vi "test图层.vi"() -> ()   [LabVIEW 2018]
doc: "This example demonstrates the use of binary morphological reconstruction in the particle analysis. The example allows you to keep the particles completely inside the ROI, completely outside the ROI or on the ROI."
uses:
  <vilib>/vision/NI_Vision_Development_Module.lvlib
panel:
  out "框组":T1(array[cluster])
  in  "单次删除":bool
  in  "Operation":T2(ring)
  out "重组图":T3(plugin-control)
  out "Image":T3(plugin-control)
  in  "Stop":bool
  # "Overview: Demonstrate the use of the Binary Morphology Reconstruction feature of Vision Development Module.\nRequirements: Vision Development Module.\nInstructions:\n1. Run the VI.\n2. Select the ROI in which you want to filter the objects. Press the <Ctrl> key to select multiple ROIs. \n3. Choose the required \"Operation\".\n  - Inner particles: Keeps all the particles completely inside the ROI.\n  - Outer particles: Keeps the particles completely outside the ROI.\n  - Boundary particles: Keeps the particles which are touching the boundary."
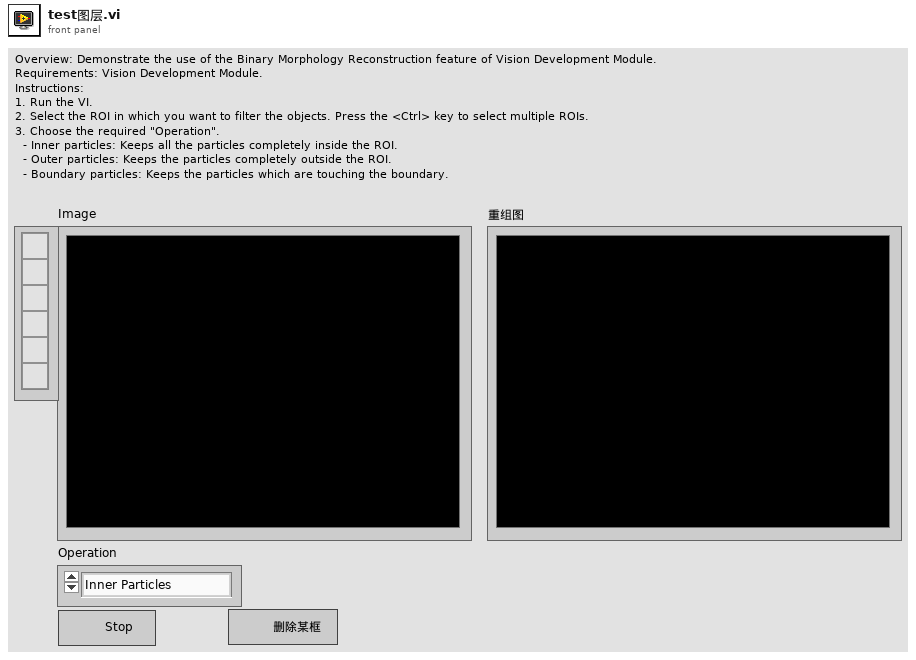
[diagram p1: front panel]
types:
  T1 = cluster{"Global Rectangle":i32[], "Contours":cluster{"Contour Type":u32, "ROI Type":u32, "Points":i32[]}[]}[]
  T2 = enum16{"Inner Particles", "Outer Particles", "Boundary Particles", "overlay rectangle"}
  T3 = typedef "IMAQ Image.ctl" = refnum<image>
  T4 = typedef "Image Type" = u32
  T5 = cluster{"Global Rectangle":i32[], "Contours":cluster{"Contour Type":u32, "ROI Type":u32, "Points":i32[]}[]}
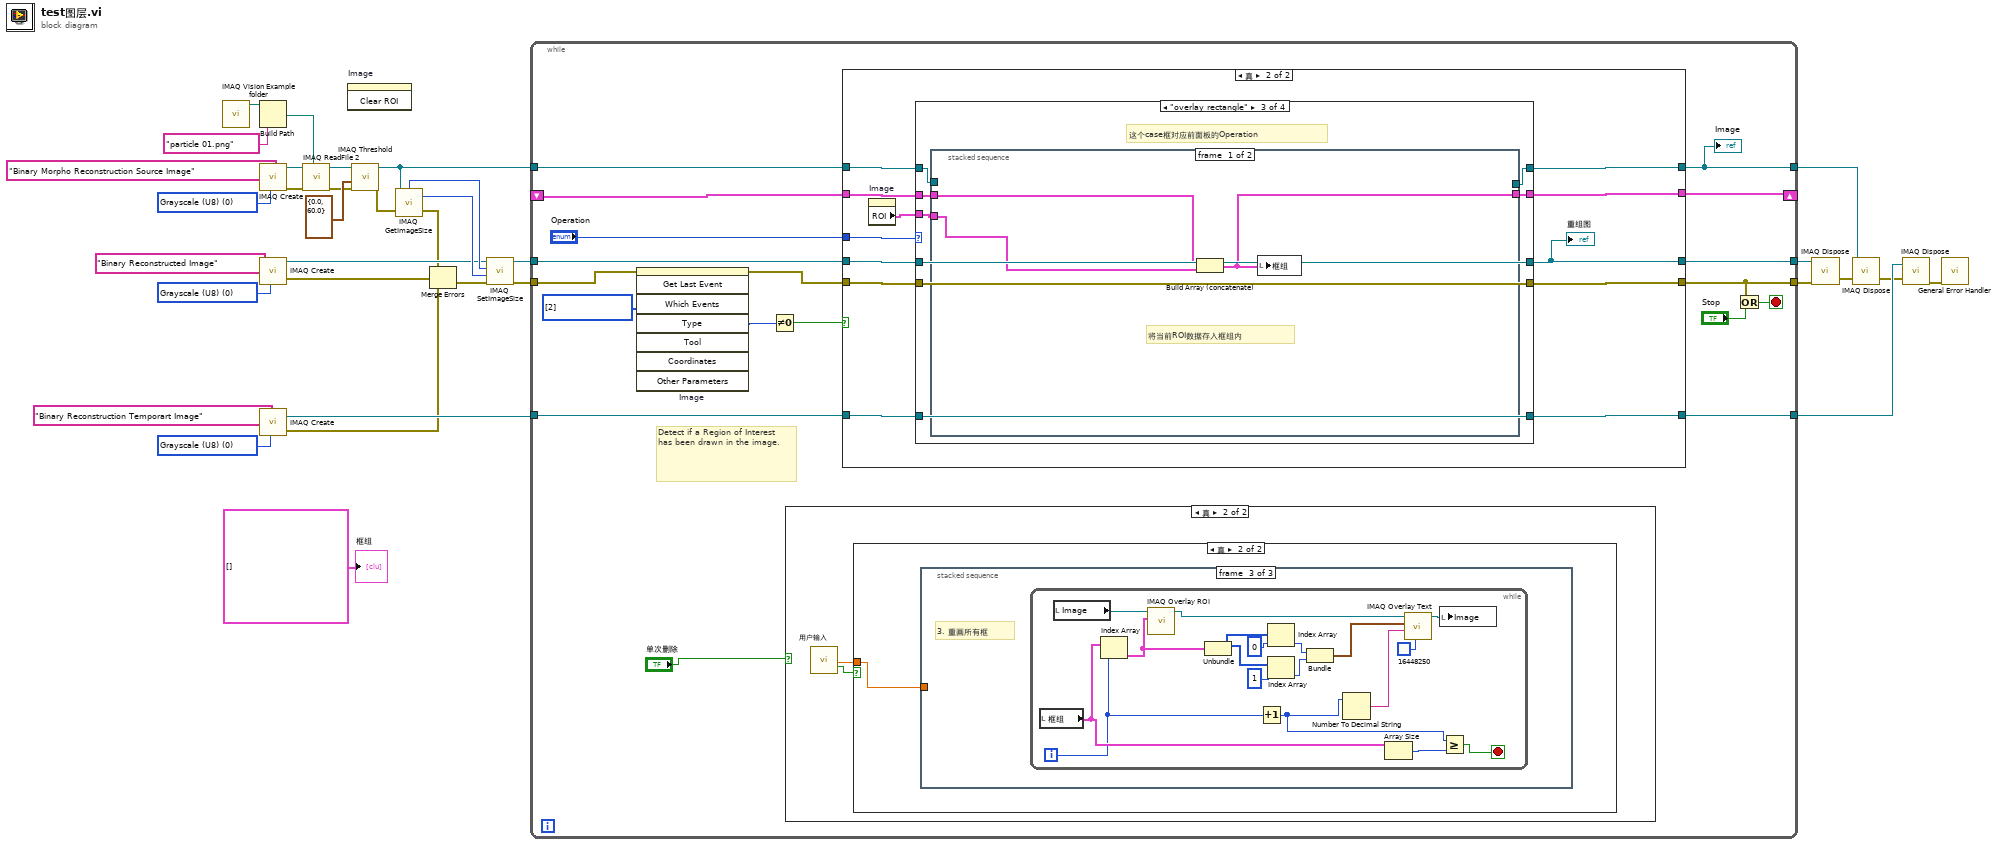
[diagram p0: block diagram]
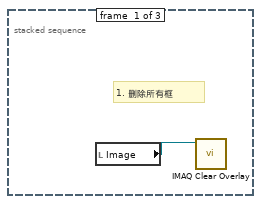
[diagram p4: hidden frame]
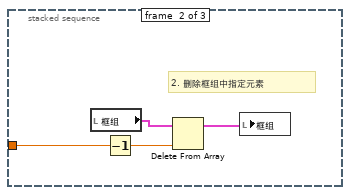
[diagram p5: hidden frame]
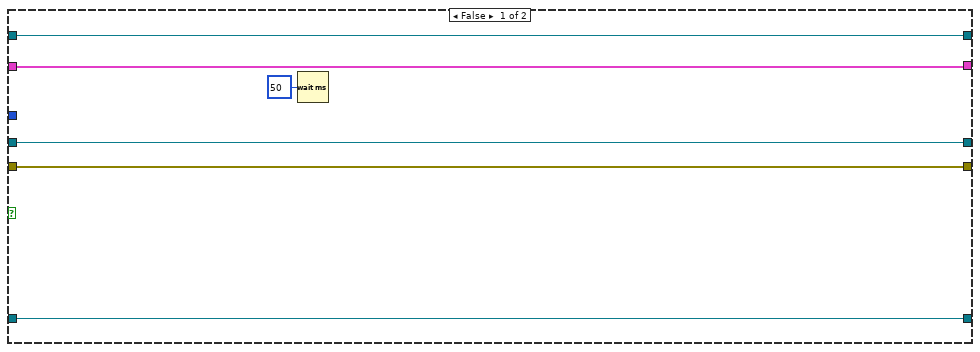
[diagram p6: hidden frame]
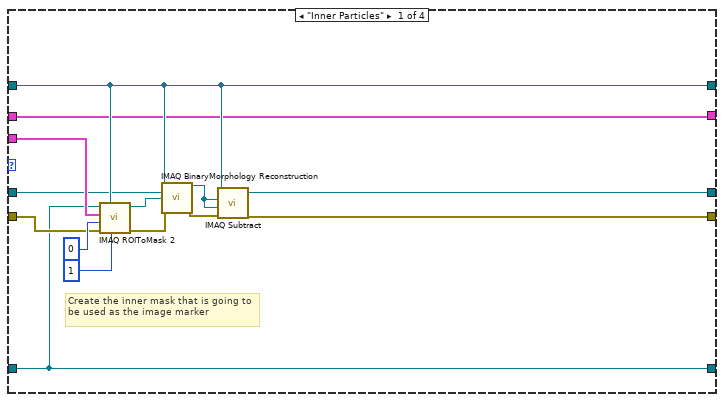
[diagram p7: hidden frame]
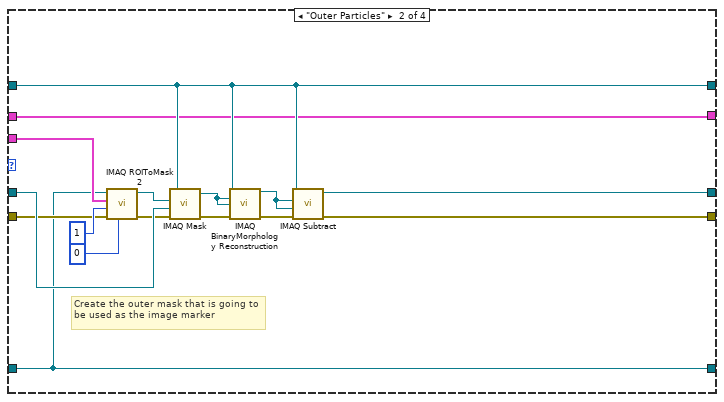
[diagram p8: hidden frame]
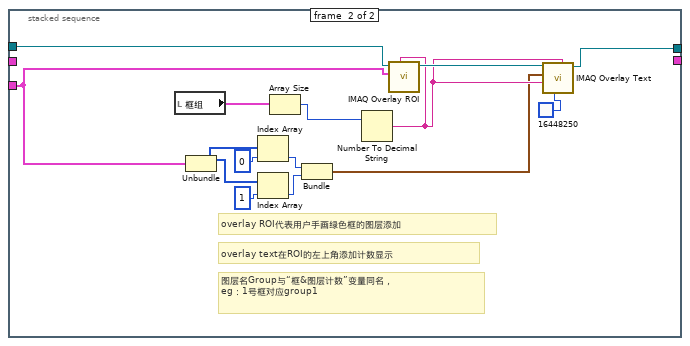
[diagram p9: hidden frame]
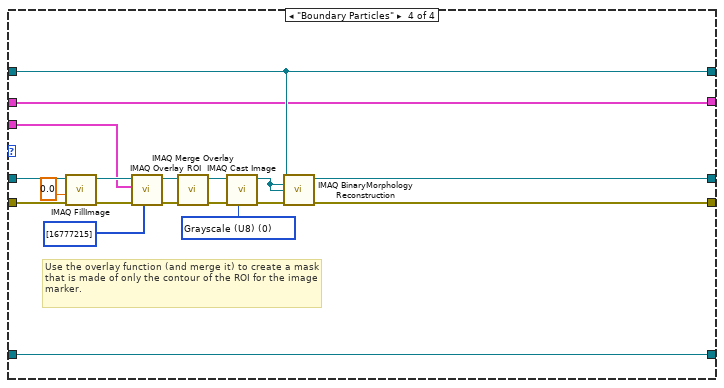
[diagram p10: hidden frame]
diagram:
  w24 = T4 0 items=["Grayscale (U8)", "Grayscale (I16)", "Grayscale (SGL)", "Complex (CSG)", "RGB (U32)", "HSL (U32)", "RGB (U64)", "Grayscale (U16)"] ("Image Type")
  w26 = T4 0 items=["Grayscale (U8)", "Grayscale (I16)", "Grayscale (SGL)", "Complex (CSG)", "RGB (U32)", "HSL (U32)", "RGB (U64)", "Grayscale (U16)"] ("Image Type")
  w27 = T4 0 items=["Grayscale (U8)", "Grayscale (I16)", "Grayscale (SGL)", "Complex (CSG)", "RGB (U32)", "HSL (U32)", "RGB (U64)", "Grayscale (U16)"] ("Image Type")
  n1 = call "IMAQ Vision Example folder.vi"() -> ("Example Image Path"=w33:path)  [unwired: 11 in]
  n2 = Build Path(base path=w33, name or relative path="particle 01.png") -> (appended path=w3:path)
  n3 = call "IMAQ Create"("Image Name"="Binary Morpho Reconstruction Source Image", "Image Type"=w26) -> ("New Image"=w30:T3, "error out"=w16:errorcluster)  [unwired: 2 in, 1 out]
  n4 = call "IMAQ Create"("Image Name"="Binary Reconstructed Image", "Image Type"=w27) -> ("New Image"=w20:T3, "error out"=w13:errorcluster)  [unwired: 2 in, 1 out]
  n5 = call "IMAQ Create"("Image Name"="Binary Reconstruction Temporart Image", "Image Type"=w24) -> ("New Image"=w21:T3, "error out"=w12:errorcluster)  [unwired: 2 in, 1 out]
  n6 = call "IMAQ ReadFile 2"("File Path"=w3, "error in (no error)"=w16, "Image"=w30) -> ("error out"=w15:errorcluster, "Image Out"=w18:T3)  [unwired: 4 in, 3 out]
  n7 = invoke on="Image" class="ImageControl" method="Clear ROI"() -> ()  [unwired: 3 in, 3 out]
  n8 = call "IMAQ Threshold"("error in (no error)"=w15, "Range"=cluster{"Lower value":sgl, "Upper value":sgl} {"Lower value"=0.0, "Upper value"=60.0}, "Image Src"=w18) -> ("error out"=w14:errorcluster, "Image Dst Out"=w2:T3)  [unwired: 3 in, 4 out]
  n9 = call "IMAQ GetImageSize"("Image"=w2, "error in (no error)"=w14) -> ("Y Resolution"=w22:i32, "X Resolution"=w23:i32, "error out"=w9:errorcluster)  [unwired: 2 out]
  n10 = Merge Errors(w9, w13, w12) -> (w11:errorcluster)
  n11 = call "IMAQ SetImageSize"("error in (no error)"=w11, "Y Resolution"=w22, "X Resolution"=w23, "Image"=w20) -> ("error out"=w10:errorcluster, "Image Out"=w19:T3)  [unwired: 1 out]
  n12 = while {
    tunnel: w2 -> [w52]
    tunnel: w19 -> [w51]
    tunnel: [w50] -> w29
    tunnel: [w39] -> w28
    tunnel: w21 -> [w49]
    tunnel: w10 -> [w45]
    tunnel: [w42] -> w7
    tunnel: [w43] -> w8
    shift-right: [w36] -> _
    shift-left: _ -> [w35]
    stop <- w40 stop-if-true
    w46 = i32[] [2] items=["No Event"=0, "Click Event"=1, "Draw Event"=2, "Size Event"=4, "Scroll Event"=5, "Double Click Event"=8] ("Which Events")
    # "Detect if a Region of Interest has been drawn in the image."
    n13 = invoke on="Image" class="ImageControl" method="Get Last Event"(error in=w45, "Which Events"=w46) -> (error out=w44:errorcluster, "Type"=w47:i32)  [unwired: 6 in, 6 out]
    n14 = Not Equal To 0?(x=w47) -> (x != 0?=w37:bool)
    n15 = case shown="真" "单次删除" {
      frame False {
      }
      frame True {
        n16 = call "用户输入"() -> ("框号"=w53:dbl, "确定"=w54:bool)  [unwired: 17 in, 1 out]
        n17 = case shown="真" w54 {
          tunnel: w53 -> [_ w55]
          frame False {
            # "用户取消操作"
          }
          frame True {
            n18 = stacked-sequence {
              tunnel: w55 -> [_ w59 _]
              frame #0 {
                # "1. 删除所有框"
                n19 = local read "Image"() -> (w56:T3)
                n20 = call "IMAQ Clear Overlay"("Image"=w56) -> ()  [unwired: 9 in, 2 out]
              }
              frame #1 {
                # "2. 删除框组中指定元素"
                n21 = local read "框组"() -> (w60:T1)
                n22 = Decrement(x=w59) -> (x-1=w58:dbl)
                n23 = Delete From Array(array=w60, index=w58) -> (array with subset deleted=w57:T1)  [unwired: 1 in, 1 out]
                n24 = local write "框组"(w57) -> ()
              }
              frame #2 {
                # "3. 重画所有框"
                n25 = while {
                  i -> [w68]
                  stop <- w77 stop-if-true
                  n26 = local read "框组"() -> (w69:T1)
                  n27 = local read "Image"() -> (w75:T3)
                  n28 = Index Array(array=w69, index=w68) -> (element=w63:T5)
                  n29 = call "IMAQ Overlay ROI"("ROI Descriptor"=w63, "Image"=w75) -> ("Image Out"=w71:T3)  [unwired: 8 in, 1 out]
                  n30 = Unbundle(w63) -> ("Global Rectangle"=w64:i32[])  [unwired: 1 out]
                  n31 = Increment(x=w68) -> (x+1=w74:i32)
                  n32 = Index Array(array=w64, index=0 ("索引")) -> (element=w65:i32)
                  n33 = Index Array(array=w64, index=1 ("索引")) -> (element=w66:i32)
                  n34 = Bundle(w65, w66) -> (w62:cluster{i32, i32})  [unwired: 1 in]
                  n35 = Number To Decimal String(number=w74) -> (decimal integer string=w72:string)  [unwired: 1 in]
                  n36 = Array Size(array=w69) -> (size(s)=w76:i32)
                  n37 = call "IMAQ Overlay Text"("Text Color (black)"=u32 16448250, "String"=w72, "Origin"=w62, "Image"=w71) -> ("Image Out"=w70:T3)  [unwired: 6 in, 1 out]
                  n38 = local write "Image"(w70) -> ()
                  n39 = Greater Or Equal?(x=w74, y=w76) -> (x >= y?=w77:bool)
                }
              }
            }
          }
        }
      }
    }
    n40 = case shown="真" w37 {
      tunnel: w52 -> [w83 w95]
      tunnel: w51 -> [w82 w94]
      tunnel: [w82 w93] -> w50
      tunnel: [w83 w92] -> w39
      tunnel: w49 -> [w80 w87]
      tunnel: "Operation" -> [_ w90]
      tunnel: w44 -> [w81 w89]
      tunnel: [w81 w88] -> w42
      tunnel: [w80 w86] -> w43
      tunnel: [w78 w85] -> w36
      tunnel: w35 -> [w78 w84]
      frame False {
        n41 = Wait (ms)(milliseconds to wait=u32 50) -> ()  [unwired: 1 out]
      }
      frame True {
        n42 = property on="Image" class="ImageControl"() -> ("ROI"=w91:T5)  [unwired: 2 in, 2 out]
        n43 = case shown="\"overlay rectangle\"" w90 {
          tunnel: w95 -> [w104 w117 w130 w166]
          tunnel: w94 -> [w102 w118 w133 w158]
          tunnel: w87 -> [w97 w111 w131 w167]
          tunnel: [w106 w120 w133 w169] -> w93
          tunnel: w91 -> [w105 w119 w128 w159]
          tunnel: [w104 w117 w129 w166] -> w92
          tunnel: w89 -> [w101 w116 w132 w157]
          tunnel: [w98 w112 w132 w168] -> w88
          tunnel: [w97 w111 w131 w167] -> w86
          tunnel: [w96 w110 w127 w151] -> w85
          tunnel: w84 -> [w96 w110 w126 w151]
          frame "Inner Particles" {
            # "Create the inner mask that is going to be used as the image marker"
            n44 = call "IMAQ ROIToMask 2"("Background Value (0)"=1, "Image Model"=w104, "error in (no error)"=w101, "Filling Value (255)"=0, "ROI Descriptor"=w105, "Image"=w97) -> ("error out"=w100:errorcluster, "Image Out"=w103:T3)  [unwired: 4 out]
            n45 = call "IMAQ BinaryMorphology Reconstruction"("Image Src"=w104, "Image Dst"=w102, "Image Marker"=w103, "error in (no error)"=w100) -> ("Image Dst Out"=w107:T3, "error out"=w99:errorcluster)  [unwired: 4 in, 6 out]
            n46 = call "IMAQ Subtract"("Image Src A"=w104, "Image Dst"=w107, "Image Src B"=w107, "error in (no error)"=w99) -> ("Image Dst Out"=w106:T3, "error out"=w98:errorcluster)  [unwired: 1 in, 2 out]
          }
          frame "Outer Particles" {
            # "Create the outer mask that is going to be used as the image marker"
            n47 = call "IMAQ ROIToMask 2"("Background Value (0)"=0, "error in (no error)"=w116, "Filling Value (255)"=1, "ROI Descriptor"=w119, "Image"=w111) -> ("error out"=w115:errorcluster, "Image Out"=w123:T3)  [unwired: 1 in, 4 out]
            n48 = call "IMAQ Mask"("error in (no error)"=w115, "Image Dst"=w118, "Image Mask"=w123, "Image Src"=w117) -> ("error out"=w114:errorcluster, "Image Dst Out"=w122:T3)  [unwired: 1 out]
            n49 = call "IMAQ BinaryMorphology Reconstruction"("Image Src"=w117, "Image Dst"=w122, "Image Marker"=w122, "error in (no error)"=w114) -> ("Image Dst Out"=w121:T3, "error out"=w113:errorcluster)  [unwired: 4 in, 6 out]
            n50 = call "IMAQ Subtract"("Image Src A"=w117, "Image Dst"=w121, "Image Src B"=w121, "error in (no error)"=w113) -> ("Image Dst Out"=w120:T3, "error out"=w112:errorcluster)  [unwired: 1 in, 2 out]
          }
          frame "overlay rectangle" {
            # "这个case框对应前面板的Operation"
            n51 = stacked-sequence {
              tunnel: w130 -> [_ w140]
              tunnel: [_ w139] -> w129
              tunnel: w128 -> [w136 w141]
              tunnel: [w134 _] -> w127
              tunnel: w126 -> [w135 _]
              frame #0 {
                # "将当前ROI数据存入框组内"
                n52 = Build Array (concatenate)(w135, w136) -> (w134:T1)
                n53 = local write "框组"(w134) -> ()
              }
              frame #1 {
                # "图层名Group与“框&图层计数”变量同名，\neg：1号框对应group1"
                # "overlay text在ROI的左上角添加计数显示"
                # "overlay ROI代表用户手画绿色框的图层添加"
                n54 = local read "框组"() -> (w146:T1)
                n55 = Unbundle(w141) -> ("Global Rectangle"=w149:i32[])  [unwired: 1 out]
                n56 = Index Array(array=w149, index=0 ("索引")) -> (element=w148:i32)
                n57 = Index Array(array=w149, index=1 ("索引")) -> (element=w147:i32)
                n58 = Array Size(array=w146) -> (size(s)=w137:i32)
                n59 = Bundle(w148, w147) -> (w138:cluster{i32, i32})  [unwired: 1 in]
                n60 = Number To Decimal String(number=w137) -> (decimal integer string=w145:string)  [unwired: 1 in]
                n61 = call "IMAQ Overlay ROI"("Group"=w145, "ROI Descriptor"=w141, "Image"=w140) -> ("Image Out"=w150:T3)  [unwired: 7 in, 1 out]
                n62 = call "IMAQ Overlay Text"("Group"=w145, "Text Color (black)"=u32 16448250, "String"=w145, "Origin"=w138, "Image"=w150) -> ("Image Out"=w139:T3)  [unwired: 5 in, 1 out]
              }
            }
          }
          frame "Boundary Particles" {
            w161 = T4 0 items=["Grayscale (U8)", "Grayscale (I16)", "Grayscale (SGL)", "Complex (CSG)", "RGB (U32)", "HSL (U32)", "RGB (U64)", "Grayscale (U16)"] ("Image Type")
            # "Use the overlay function (and merge it) to create a mask that is made of only the contour of the ROI for the image marker."
            n63 = call "IMAQ FillImage"("error in (no error)"=w157, "Pixel Value (U8, U16, I16, Float)"=sgl 0.0, "Image"=w158) -> ("error out"=w156:errorcluster, "Image Out"=w164:T3)  [unwired: 4 in, 3 out]
            n64 = call "IMAQ Overlay ROI"("Colors (Green)"=u32[] [16777215], "error in (no error)"=w156, "ROI Descriptor"=w159, "Image"=w164) -> ("error out"=w155:errorcluster, "Image Out"=w165:T3)  [unwired: 2 in, 4 out]
            n65 = call "IMAQ Merge Overlay"("error in (no error)"=w155, "Image Src"=w165) -> ("error out"=w154:errorcluster, "Image Dst Out"=w162:T3)  [unwired: 3 in, 5 out]
            n66 = call "IMAQ Cast Image"("Image Type"=w161, "error in (no error)"=w154, "Image Src"=w162) -> ("error out"=w153:errorcluster, "Image Dst Out"=w152:T3)  [unwired: 3 in, 4 out]
            n67 = call "IMAQ BinaryMorphology Reconstruction"("Image Src"=w166, "Image Dst"=w152, "Image Marker"=w152, "error in (no error)"=w153) -> ("Image Dst Out"=w169:T3, "error out"=w168:errorcluster)  [unwired: 4 in, 6 out]
          }
        }
        "重组图" <- w93
      }
    }
    "Image" <- w39
    n68 = Or(x=w42, y="Stop") -> (x .or. y?=w40:bool)
  }
  n69 = call "IMAQ Dispose"("Image"=w29, "error in (no error)"=w7) -> ("error out"=w6:errorcluster)  [unwired: 1 in, 3 out]
  n70 = call "IMAQ Dispose"("Image"=w28, "error in (no error)"=w6) -> ("error out"=w5:errorcluster)  [unwired: 1 in, 3 out]
  n71 = call "IMAQ Dispose"("Image"=w8, "error in (no error)"=w5) -> ("error out"=w4:errorcluster)  [unwired: 1 in, 3 out]
  n72 = call <vilib>:"General Error Handler.vi"("error in (no error)"=w4) -> ()  [unwired: 10 in, 5 out]
  "框组" <- T1 [] ("框组")
